vi "To True Color Image.vi"(8 "error in (no error)":errorcluster, 11 "Image":T1) -> (0 "error out":errorcluster, 3 "True Color Image":T1)   [LabVIEW 2020, in "G-Image.lvlib"]
doc: "Converts the input image to a true color image.\n\n- 8-bit images without a mask are converted to 24-bit RGB.\n- 8-bit and 24-bit images with a mask are converted to 32-bit ARGB, where the mask is applied to the alpha channel."
uses:
  G-Image.lvlib
  <vilib>/picture/picture.llb/imagedata.ctl
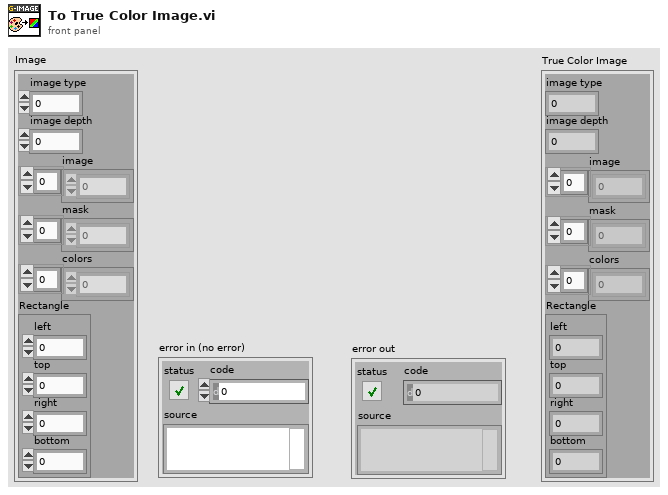
[diagram p1: front panel]
types:
  T1 = typedef "imagedata.ctl" = cluster{"image type":i32, "image depth":i32, "image":u8[], "mask":u8[], "colors":u32[], "Rectangle":cluster{"left":i16, "top":i16, "right":i16, "bottom":i16}}
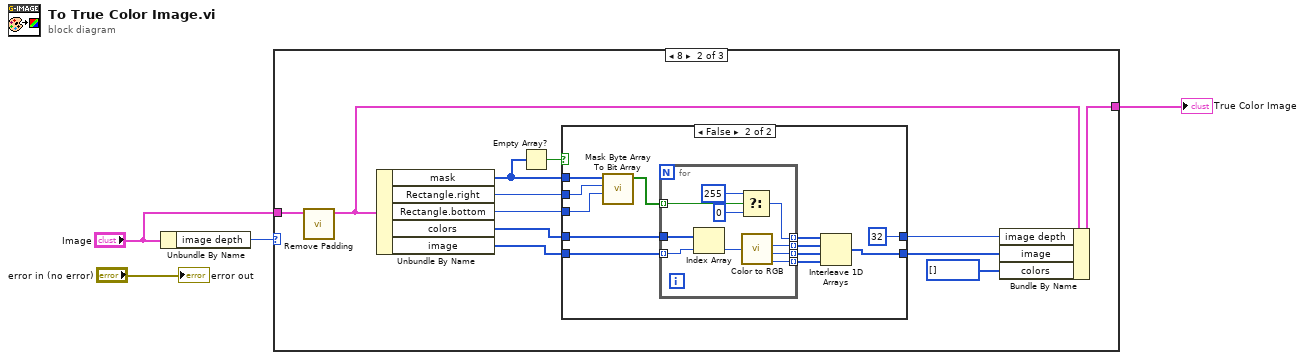
[diagram p0: block diagram]
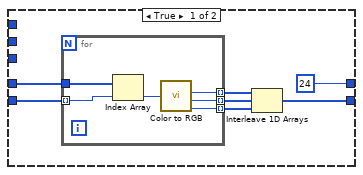
[diagram p3: hidden frame]
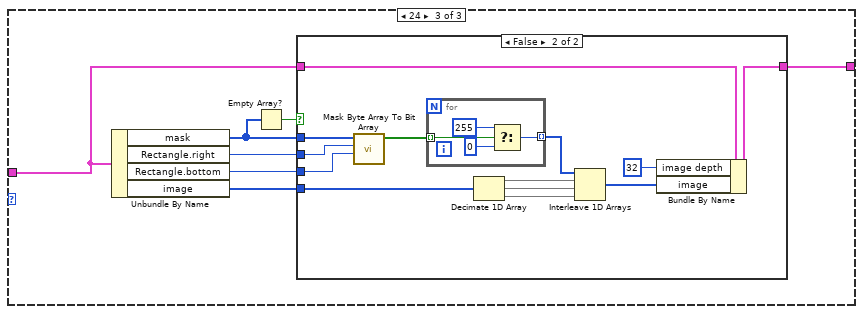
[diagram p4: hidden frame]
diagram:
  n1 = Unbundle By Name("Image") -> ("image depth"=w3:i32)
  n2 = case shown="8" w3 {
    tunnel: [w5 w10 w53] -> w1
    tunnel: "Image" -> [w5 w14 w54]
    frame Default {
    }
    frame 8 {
      n3 = call "Remove Padding.vi"("Image"=w14) -> ("Image Out"=w6:T1)  [unwired: 9 in, 1 out]
      n4 = Unbundle By Name(w6) -> ("mask"=w7:u8[], "Rectangle.right"=w9:i16, "Rectangle.bottom"=w8:i16, "colors"=w15:u32[], "image"=w16:u8[])
      n5 = Empty Array?(array=w7) -> (empty?=w17:bool)
      n6 = case shown="False" w17 {
        tunnel: w16 -> [w24 w35]
        tunnel: w15 -> [w23 w42]
        tunnel: w7 -> [_ w34]
        tunnel: [24 32] -> w13
        tunnel: [w19 w38] -> w12
        tunnel: w9 -> [_ w33]
        tunnel: w8 -> [_ w32]
        frame True {
          n7 = for {
            tunnel: w24 -> [w29] mode=indexing
            tunnel: w23 -> [w30]
            tunnel: [w27] -> w22 mode=indexing
            tunnel: [w26] -> w21 mode=indexing
            tunnel: [w25] -> w20 mode=indexing
            n8 = Index Array(array=w30, index=w29) -> (element=w28:u32)
            n9 = call <vilib>:"Color to RGB.vi"("Color"=w28) -> ("R"=w27:u8, "G"=w26:u8, "B"=w25:u8)  [unwired: 1 out]
          }
          n10 = Interleave 1D Arrays(w22, w21, w20) -> (w19:u8[])
        }
        frame False {
          n11 = call "Mask Byte Array To Bit Array.vi"("Height"=w32, "Width"=w33, "Image Mask"=w34) -> ("Boolean Mask"=w31:bool[])  [unwired: 8 in]
          n12 = for {
            tunnel: w35 -> [w51] mode=indexing
            tunnel: w42 -> [w52]
            tunnel: [w49] -> w41 mode=indexing
            tunnel: [w48] -> w40 mode=indexing
            tunnel: [w47] -> w39 mode=indexing
            tunnel: w31 -> [w46] mode=indexing
            tunnel: [w43] -> w36 mode=indexing
            n13 = Index Array(array=w52, index=w51) -> (element=w50:u32)
            n14 = Select(t=u8 255, s=w46, f=u8 0) -> (s? t:f=w43:u8)
            n15 = call <vilib>:"Color to RGB.vi"("Color"=w50) -> ("R"=w49:u8, "G"=w48:u8, "B"=w47:u8)  [unwired: 1 out]
          }
          n16 = Interleave 1D Arrays(w36, w41, w40, w39) -> (w38:u8[])
        }
      }
      n17 = Bundle By Name(cluster=w6, "image depth"=w13, "image"=w12, "colors"=u32[] []) -> (w10:T1)
    }
    frame 24 {
      n18 = Unbundle By Name(w54) -> ("mask"=w55:u8[], "Rectangle.right"=w57:i16, "Rectangle.bottom"=w56:i16, "image"=w58:u8[])
      n19 = Empty Array?(array=w55) -> (empty?=w59:bool)
      n20 = case shown="False" w59 {
        tunnel: w58 -> [_ w65]
        tunnel: w55 -> [_ w72]
        tunnel: w57 -> [_ w71]
        tunnel: w56 -> [_ w70]
        tunnel: [w60 w61] -> w53
        tunnel: w54 -> [w60 w68]
        frame True {
        }
        frame False {
          n21 = call "Mask Byte Array To Bit Array.vi"("Height"=w70, "Width"=w71, "Image Mask"=w72) -> ("Boolean Mask"=w69:bool[])  [unwired: 8 in]
          n22 = for {
            tunnel: w69 -> [w77] mode=indexing
            tunnel: [w74] -> w73 mode=indexing
            n23 = Select(t=u8 255, s=w77, f=u8 0) -> (s? t:f=w74:u8)
          }
          n24 = Decimate 1D Array(w65) -> (w64:u8[], w63:u8[], w62:u8[])
          n25 = Interleave 1D Arrays(w73, w64, w63, w62) -> (w66:u8[])
          n26 = Bundle By Name(cluster=w68, "image depth"=32, "image"=w66) -> (w61:T1)
        }
      }
    }
  }
  "True Color Image" <- w1
  "error out" <- "error in (no error)"
